vi "SingleLayerReport.vi"(0 "IP address":string="192.168.1.214", 5 "LayerID under test":u32 format="%x", 7 "All ID list":u32[](array[numeric]) format="%x", 9 "Report folder path":path, 11 "process":string) -> (4 "Layer Report file path":path, 8 "Test OK?":bool, 10 "Report out":string, 15 "error out":errorcluster)   [LabVIEW 2015, in "VIPM2.lvlib"]
uses:
  VIPM2.lvlib
panel:
  in  "TDCValues":i32=5
  out "STATUS MONITOR":string="CLOSING TCP/IP CONNECTION"
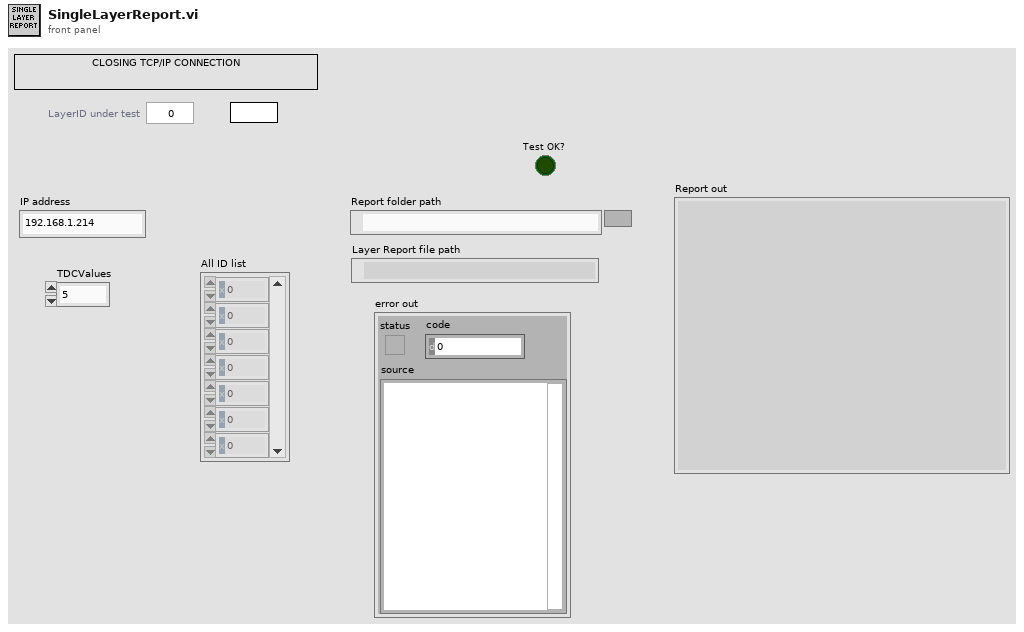
[diagram p1: front panel]
types:
  T1 = enum16{"open", "replace", "create", "open or create", "replace or create", "replace or create with confirmation"}
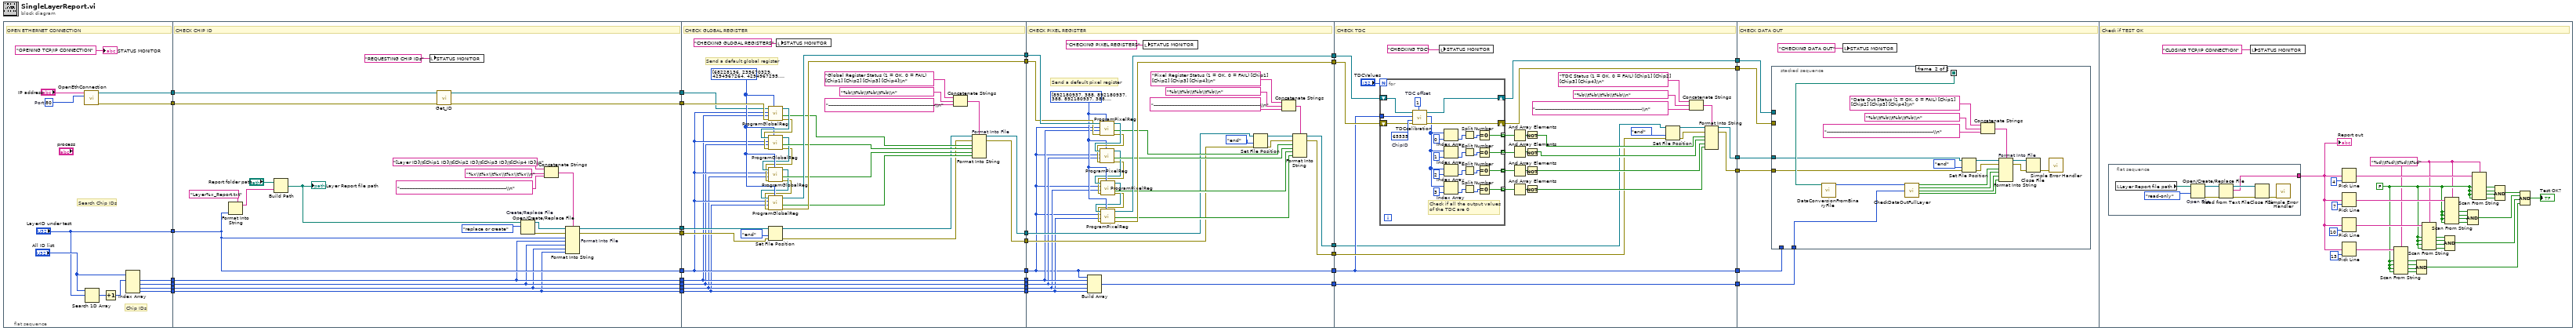
[diagram p0: block diagram]
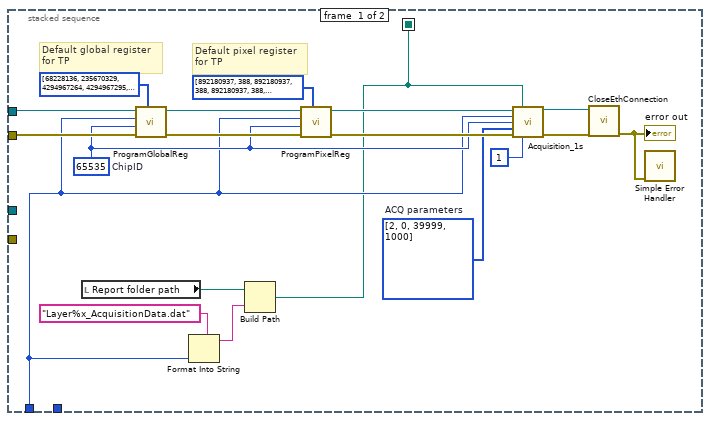
[diagram p2: hidden frame]
diagram:
  n1 = flat-sequence {
    tunnel: [w47] -> w7
    tunnel: [w46] -> w6
    tunnel: ["LayerID under test"] -> w5
    tunnel: [w41] -> w4
    tunnel: [w40] -> w3
    tunnel: [w39] -> w2
    tunnel: [w38] -> w1
    tunnel: w7 -> [w54]
    tunnel: [w52] -> w37
    tunnel: w6 -> [w53]
    tunnel: [w51] -> w36
    tunnel: [w59] -> w29
    tunnel: [w58] -> w28
    tunnel: [w57] -> w27
    tunnel: [w56] -> w26
    tunnel: [w55] -> w25
    tunnel: [w61] -> w24
    tunnel: [w60] -> w23
    tunnel: w5 -> [w59]
    tunnel: w4 -> [w58]
    tunnel: w3 -> [w57]
    tunnel: w2 -> [w56]
    tunnel: w1 -> [w55]
    tunnel: w37 -> [w85]
    tunnel: [w105] -> w35
    tunnel: w36 -> [w104]
    tunnel: [w103] -> w34
    tunnel: w29 -> [w80]
    tunnel: w28 -> [w79]
    tunnel: w27 -> [w78]
    tunnel: w26 -> [w77]
    tunnel: w25 -> [w76]
    tunnel: w24 -> [w84]
    tunnel: w23 -> [w83]
    tunnel: [w80] -> w22
    tunnel: [w79] -> w21
    tunnel: [w78] -> w20
    tunnel: [w77] -> w19
    tunnel: [w76] -> w18
    tunnel: [w75] -> w17
    tunnel: [w74] -> w16
    tunnel: w35 -> [w138]
    tunnel: [w137] -> w33
    tunnel: w34 -> [w134]
    tunnel: [w136] -> w32
    tunnel: w22 -> [w106]
    tunnel: w21 -> [w111]
    tunnel: w20 -> [w110]
    tunnel: w19 -> [w109]
    tunnel: w18 -> [w108]
    tunnel: w17 -> [w115]
    tunnel: w16 -> [w114]
    tunnel: [w106] -> w15
    tunnel: [w113] -> w14
    tunnel: [w112] -> w13
    tunnel: [w107] -> w9
    tunnel: w33 -> [w169]
    tunnel: [w168] -> w31
    tunnel: w32 -> [w167]
    tunnel: [w166] -> w30
    tunnel: w15 -> [w143]
    tunnel: w14 -> [w142]
    tunnel: w13 -> [w144]
    tunnel: [w143] -> w12
    tunnel: [w141] -> w11
    tunnel: [w140] -> w10
    tunnel: w9 -> [w139]
    tunnel: [w139] -> w8
    tunnel: w31 -> [w197]
    tunnel: w30 -> [w199]
    tunnel: w12 -> [w198]
    tunnel: w11 -> [w196]
    tunnel: w10 -> [w195]
    tunnel: w8 -> [w194]
    frame #0 {
      w49 = u16 80  # Port
      # "Chip IDs"
      # "Search Chip IDs"
      # "OPEN ETHERNET CONNECTION"
      n2 = call "OpenEthConnection.vi"("Port"=w49, "IP address"="IP address") -> ("error out"=w46:errorcluster, "connection ID out"=w47:refnum<k5>)  [unwired: 7 in, 1 out]
      n3 = Search 1D Array(1D array="All ID list", element="LayerID under test") -> (index of element=w44:i32)  [unwired: 1 in]
      n4 = Increment(x=w44) -> (x+1=w45:i32)
      n5 = Index Array "Index Array"(array="All ID list", index #1=w45) -> (element #1=w41:u32, element #2=w40:u32, element #3=w39:u32, element #4=w38:u32)  [unwired: 3 in]
      "STATUS MONITOR" <- "OPENING TCP/IP CONNECTION" ("STATUS MONITOR")
    }
    frame #1 {
      # "CHECK CHIP ID"
      n6 = Format Into String(format string="Layer%x_Report.txt", w59) -> (resulting string=w63:string)  [unwired: 2 in, 1 out]
      n7 = Build Path(base path="Report folder path", name or relative path=w63) -> (appended path=w72:path)
      "Layer Report file path" <- w72
      n8 = local write "STATUS MONITOR"("REQUESTING CHIP IDs" ("STATUS MONITOR")) -> ()
      n9 = call "Get_ID.vi"("error in (no error)"=w53, "connection ID"=w54) -> ("error out"=w51:errorcluster, "connection ID out"=w52:refnum<k5>)  [unwired: 6 in, 2 out]
      n10 = Open/Create/Replace File "Create/Replace File"(file path (use dialog)=w72, operation (0:open)=T1."replace or create") -> (refnum out=w70:refnum<file>, error out=w65:errorcluster)  [unwired: 4 in, 1 out]
      n11 = Concatenate Strings "Concatenate Strings"("[Layer ID]\\t[Chip1 ID]\\t[Chip2 ID]\\t[Chip3 ID]\\t[Chip4 ID]\\n" ("format string"), "%x\\t%x\\t%x\\t%x\\t%x\\n" ("format string"), "--------------------------------------------------------------------\\n" ("format string")) -> (w66:string)
      n12 = Format Into String "Format Into File"(format string=w66, initial string=w70, error in=w65, w59, w58, w57, w56, w55) -> (resulting string=w61:refnum<file>, error out=w60:errorcluster)
    }
    frame #2 {
      w90 = u32[] [68228136, 235670329, 4294967264, 4294967295, 4294967295, 511] ("DefaultGlobal Reg_TP")
      # "Send a default global register"
      # "CHECK GLOBAL REGISTER"
      n13 = call "ProgramGlobalReg.vi"("Global Reg"=w90, "error in (no error)"=w104, "ChipID"=w79, "LayerID"=w80, "connection ID"=w85) -> ("error out"=w93:errorcluster, "OK?"=w91:bool, "connection ID out"=w101:refnum<k5>)  [unwired: 2 in, 2 out]
      n14 = call "ProgramGlobalReg.vi"("Global Reg"=w90, "error in (no error)"=w93, "ChipID"=w78, "LayerID"=w80, "connection ID"=w101) -> ("error out"=w87:errorcluster, "OK?"=w96:bool, "connection ID out"=w89:refnum<k5>)  [unwired: 2 in, 2 out]
      n15 = Set File Position(refnum=w84, from (0:start)=enum16{"start", "end", "current"}."end", error in=w83) -> (refnum out=w82:refnum<file>, error out=w81:errorcluster)  [unwired: 1 in]
      n16 = call "ProgramGlobalReg.vi"("Global Reg"=w90, "error in (no error)"=w87, "ChipID"=w77, "LayerID"=w80, "connection ID"=w89) -> ("error out"=w86:errorcluster, "OK?"=w95:bool, "connection ID out"=w88:refnum<k5>)  [unwired: 2 in, 2 out]
      n17 = call "ProgramGlobalReg.vi"("Global Reg"=w90, "error in (no error)"=w86, "ChipID"=w76, "LayerID"=w80, "connection ID"=w88) -> ("error out"=w103:errorcluster, "OK?"=w94:bool, "connection ID out"=w105:refnum<k5>)  [unwired: 2 in, 2 out]
      n18 = local write "STATUS MONITOR"("CHECKING GLOGAL REGISTERS" ("STATUS MONITOR")) -> ()
      n19 = Concatenate Strings "Concatenate Strings"("Global Register Status (1 = OK, 0 = FAIL) [Chip1] [Chip2] [Chip3] [Chip4]\\n" ("format string"), "%b\\t%b\\t%b\\t%b\\n" ("format string"), "--------------------------------------------------------------------\\n" ("format string")) -> (w99:string)
      n20 = Format Into String "Format Into File"(format string=w99, initial string=w82, error in=w81, w91, w96, w95, w94) -> (resulting string=w75:refnum<file>, error out=w74:errorcluster)
    }
    frame #3 {
      w121 = u32[] [892180937, 388, 892180937, 388, 892180937, 388, 892180937, 388, 892180937, 388, 892180937, 388, 892180937, 388, 892180937, 388, 892180937, 388, 892180937, 388, 892180937, 388, 892180937, 388, 892180937, 388, 892180937, 388, 892180937, 388, 892180937, 388, 892180937, 388, 892180937, 388, 892180937, 388, 892180937, 388, 892180937, 388, 892180937, 388, 892180937, 388, 892180937, 388, 892180937, 388, 892180937, 388, 892180937, 388, 892180937, 388, 892180937, 388, 892180937, 388, 892180937, 388, 892180937, 388, 892180937, 388, 1092475113, 180, 892180937, 388, 892180937, 388, 892180937, 388, 892180937, 388, 892180937, 388, 892180937, 388, 892180937, 388, 892180937, 388, 892180937, 388, 892180937, 388, 892180937, 388, 892180937, 388, 892180937, 388, 892180937, 388, 892180937, 388, 892180937, 388, 892180937, 388, 892180937, 388, 892180937, 388, 892180937, 388, 892180937, 388, 892180937, 388, 892180937, 388, 892180937, 388, 892180937, 388, 892180937, 388, 892180937, 388, 892180937, 388, 892180937, 388, 892180937, 388, 892180937, 388, 892180937, 388, 892180937, 388, 892180937, 388, 892180937, 388, 892180937, 388, 892180937, 388, 892180937, 388, 892180937, 388, 892180937, 388, 892180937, 388, 892180937, 388, 892180937, 388, 892180937, 388, 892180937, 388, 892180937, 388, 892180937, 388, 892180937, 388, 892180937, 388, 892180937, 388, 892180937, 388, 892180937, 388, 892180937, 388, 892180937, 388, 892180937, 388, 892180937, 388, 892180937, 388, 892180937, 388, 892180937, 388, 892180937, 388, 892180937, 388, 892180937, 388, 892180937, 388, 892180937, 388, 892180937, 388, 892180937, 388] ("DefaultPixel Register Array_TP")
      # "Send a default pixel register"
      # "CHECK PIXEL REGISTER"
      n21 = Build Array "Build Array"(w106, w111, w110, w109, w108) -> (w107:u32[])
      n22 = call "ProgramPixelReg.vi"("Pixel Register"=w121, "error in (no error)"=w134, "ChipID"=w111, "LayerID"=w106, "connection ID"=w138) -> ("error out"=w126:errorcluster, "OK?"=w122:bool, "connection ID out"=w133:refnum<k5>)  [unwired: 2 in, 2 out]
      n23 = call "ProgramPixelReg.vi"("Pixel Register"=w121, "error in (no error)"=w126, "ChipID"=w110, "LayerID"=w106, "connection ID"=w133) -> ("error out"=w118:errorcluster, "OK?"=w129:bool, "connection ID out"=w120:refnum<k5>)  [unwired: 2 in, 2 out]
      n24 = call "ProgramPixelReg.vi"("Pixel Register"=w121, "error in (no error)"=w118, "ChipID"=w109, "LayerID"=w106, "connection ID"=w120) -> ("error out"=w117:errorcluster, "OK?"=w128:bool, "connection ID out"=w119:refnum<k5>)  [unwired: 2 in, 2 out]
      n25 = call "ProgramPixelReg.vi"("Pixel Register"=w121, "error in (no error)"=w117, "ChipID"=w108, "LayerID"=w106, "connection ID"=w119) -> ("error out"=w136:errorcluster, "OK?"=w127:bool, "connection ID out"=w137:refnum<k5>)  [unwired: 2 in, 2 out]
      n26 = local write "STATUS MONITOR"("CHECKING PIXEL REGISTERS" ("STATUS MONITOR")) -> ()
      n27 = Set File Position(refnum=w115, from (0:start)=enum16{"start", "end", "current"}."end", error in=w114) -> (refnum out=w124:refnum<file>, error out=w116:errorcluster)  [unwired: 1 in]
      n28 = Concatenate Strings("Pixel Register Status (1 = OK, 0 = FAIL) [Chip1] [Chip2] [Chip3] [Chip4]\\n" ("format string"), "%b\\t%b\\t%b\\t%b\\n" ("format string"), "--------------------------------------------------------------------\\n" ("format string")) -> (w123:string)
      n29 = Format Into String(format string=w123, initial string=w124, error in=w116, w122, w129, w128, w127) -> (resulting string=w113:refnum<file>, error out=w112:errorcluster)
    }
    frame #4 {
      # "CHECK TDC"
      n30 = for {
        N: "TDCValues" -> [_]
        tunnel: w143 -> [w192]
        shift-right: [w189] -> w166
        shift-left: w167 -> [w190]
        shift-right: [w170] -> w168
        shift-left: w169 -> [w171]
        tunnel: [w175] -> w163 mode=indexing
        tunnel: [w174] -> w162 mode=indexing
        tunnel: [w173] -> w161 mode=indexing
        tunnel: [w172] -> w160 mode=indexing
        w191 = u32 65535  # ChipID
        w193 = u32 1  # TDC offset
        # "Check if all the output values\nof the TDC are 0"
        n31 = call "TDCcalibration.vi"("TDC offset"=w193, "error in (no error)"=w190, "ChipID"=w191, "LayerID"=w192, "connection ID"=w171) -> ("error out"=w189:errorcluster, "TDC calibration data"=w188:u32[], "connection ID out"=w170:refnum<k5>)  [unwired: 3 in, 1 out]
        n32 = Index Array(array=w188, index=0) -> (element=w183:u32)
        n33 = Index Array(array=w188, index=1) -> (element=w178:u32)
        n34 = Index Array(array=w188, index=2) -> (element=w177:u32)
        n35 = Index Array(array=w188, index=3) -> (element=w176:u32)
        n36 = Split Number(x=w183) -> (lo(x)=w182:u16)  [unwired: 1 out]
        n37 = Split Number(x=w178) -> (lo(x)=w181:u16)  [unwired: 1 out]
        n38 = Split Number(x=w177) -> (lo(x)=w180:u16)  [unwired: 1 out]
        n39 = Split Number(x=w176) -> (lo(x)=w179:u16)  [unwired: 1 out]
        n40 = Equal To 0?(x=w182) -> (x = 0?=w175:bool)
        n41 = Equal To 0?(x=w181) -> (x = 0?=w174:bool)
        n42 = Equal To 0?(x=w180) -> (x = 0?=w173:bool)
        n43 = Equal To 0?(x=w179) -> (x = 0?=w172:bool)
      }
      n44 = local write "STATUS MONITOR"("CHECKING TDC" ("STATUS MONITOR")) -> ()
      n45 = And Array Elements(Boolean array=w163) -> (logical AND=w154:bool)
      n46 = And Array Elements(Boolean array=w162) -> (logical AND=w153:bool)
      n47 = And Array Elements(Boolean array=w161) -> (logical AND=w152:bool)
      n48 = And Array Elements(Boolean array=w160) -> (logical AND=w151:bool)
      n49 = Not(x=w154) -> (.not. x?=w150:bool)
      n50 = Not(x=w153) -> (.not. x?=w149:bool)
      n51 = Not(x=w152) -> (.not. x?=w148:bool)
      n52 = Not(x=w151) -> (.not. x?=w147:bool)
      n53 = Set File Position(refnum=w142, from (0:start)=enum16{"start", "end", "current"}."end", error in=w144) -> (refnum out=w156:refnum<file>, error out=w146:errorcluster)  [unwired: 1 in]
      n54 = Concatenate Strings("TDC Status (1 = OK, 0 = FAIL) [Chip1] [Chip2] [Chip3] [Chip4]\\n" ("format string"), "%b\\t%b\\t%b\\t%b\\n" ("format string"), "--------------------------------------------------------------------\\n" ("format string")) -> (w155:string)
      n55 = Format Into String(format string=w155, initial string=w156, error in=w146, w150, w149, w148, w147) -> (resulting string=w141:refnum<file>, error out=w140:errorcluster)
    }
    frame #5 {
      # "CHECK DATA OUT"
      n56 = stacked-sequence {
        seq-local: [w204 _] -> [_ w223]
        tunnel: w199 -> [w219 _]
        tunnel: w198 -> [w205 _]
        tunnel: w197 -> [w209 _]
        tunnel: w195 -> [_ w222]
        tunnel: w196 -> [_ w221]
        tunnel: w194 -> [_ w220]
        frame #0 {
          w211 = u32[] [2, 0, 39999, 1000]  # ACQ parameters
          w212 = u32 65535  # ChipID
          # "Default pixel register \nfor TP"
          # "Default global register \nfor TP"
          n57 = local read "Report folder path"() -> (w207:path)
          n58 = call "ProgramGlobalReg.vi"("Global Reg"=u32[] [68228136, 235670329, 4294967264, 4294967295, 4294967295, 511] ("DefaultGlobal Reg_TP"), "error in (no error)"=w219, "ChipID"=w212, "LayerID"=w205, "connection ID"=w209) -> ("error out"=w216:errorcluster, "connection ID out"=w217:refnum<k5>)  [unwired: 2 in, 3 out]
          n59 = Format Into String(format string="Layer%x_AcquisitionData.dat", w205) -> (resulting string=w206:string)  [unwired: 2 in, 1 out]
          n60 = Build Path(base path=w207, name or relative path=w206) -> (appended path=w204:path)
          n61 = call "ProgramPixelReg.vi"("Pixel Register"=u32[] [892180937, 388, 892180937, 388, 892180937, 388, 892180937, 388, 892180937, 388, 892180937, 388, 892180937, 388, 892180937, 388, 892180937, 388, 892180937, 388, 892180937, 388, 892180937, 388, 892180937, 388, 892180937, 388, 892180937, 388, 892180937, 388, 892180937, 388, 892180937, 388, 892180937, 388, 892180937, 388, 892180937, 388, 892180937, 388, 892180937, 388, 892180937, 388, 892180937, 388, 892180937, 388, 892180937, 388, 892180937, 388, 892180937, 388, 892180937, 388, 892180937, 388, 892180937, 388, 892180937, 388, 1092475113, 180, 892180937, 388, 892180937, 388, 892180937, 388, 892180937, 388, 892180937, 388, 892180937, 388, 892180937, 388, 892180937, 388, 892180937, 388, 892180937, 388, 892180937, 388, 892180937, 388, 892180937, 388, 892180937, 388, 892180937, 388, 892180937, 388, 892180937, 388, 892180937, 388, 892180937, 388, 892180937, 388, 892180937, 388, 892180937, 388, 892180937, 388, 892180937, 388, 892180937, 388, 892180937, 388, 892180937, 388, 892180937, 388, 892180937, 388, 892180937, 388, 892180937, 388, 892180937, 388, 892180937, 388, 892180937, 388, 892180937, 388, 892180937, 388, 892180937, 388, 892180937, 388, 892180937, 388, 892180937, 388, 892180937, 388, 892180937, 388, 892180937, 388, 892180937, 388, 892180937, 388, 892180937, 388, 892180937, 388, 892180937, 388, 892180937, 388, 892180937, 388, 892180937, 388, 892180937, 388, 892180937, 388, 892180937, 388, 892180937, 388, 892180937, 388, 892180937, 388, 892180937, 388, 892180937, 388, 892180937, 388, 892180937, 388, 892180937, 388, 892180937, 388, 892180937, 388, 892180937, 388, 892180937, 388] ("DefaultPixel Register Array_TP"), "error in (no error)"=w216, "ChipID"=w212, "LayerID"=w205, "connection ID"=w217) -> ("error out"=w214:errorcluster, "connection ID out"=w213:refnum<k5>)  [unwired: 2 in, 3 out]
          n62 = call "Acquisition_1s.vi"("connection ID"=w213, "File ACQ data"=w204, "LayerID"=w205, "ChipID"=w212, "ACQ parameters"=w211, "error in (no error)"=w214, "Acquisition time (s)"=u32 1) -> ("connection ID out"=w203:refnum<k5>, "error out"=w202:errorcluster)  [unwired: 4 in, 3 out]
          n63 = call "CloseEthConnection.vi"("error in (no error)"=w202, "connection ID"=w203) -> ("error out"=w201:errorcluster)  [unwired: 9 in]
          "error out" <- w201
          n64 = call <vilib>:"Simple Error Handler.vi"("error in (no error)"=w201) -> ()  [unwired: 4 in, 5 out]
        }
        frame #1 {
          n65 = call "DataConversionFromBinaryFile.vi"("file (use dialog)"=w223) -> ("Output Array"=w238:u32[])  [unwired: 8 in]
          n66 = call "CheckDataOutFullLayer.vi"("InputEventWord"=w238, "ID list"=w220) -> ("DataChip1 OK?"=w230:bool, "DataChip2 OK?"=w229:bool, "DataChip3 OK?"=w228:bool, "DataChip4 OK?"=w227:bool)  [unwired: 10 in]
          n67 = Set File Position(refnum=w221, from (0:start)=enum16{"start", "end", "current"}."end", error in=w222) -> (refnum out=w232:refnum<file>, error out=w226:errorcluster)  [unwired: 1 in]
          n68 = Concatenate Strings "Concatenate Strings"("Data Out Status (1 = OK, 0 = FAIL) [Chip1] [Chip2] [Chip3] [Chip4]\\n" ("format string"), "%b\\t%b\\t%b\\t%b\\n" ("format string"), "--------------------------------------------------------------------\\n" ("format string")) -> (w231:string)
          n69 = Format Into String "Format Into File"(format string=w231, initial string=w232, error in=w226, w230, w229, w228, w227) -> (resulting string=w234:refnum<file>, error out=w225:errorcluster)
          n70 = Close File(refnum=w234, error in=w225) -> (error out=w224:errorcluster)  [unwired: 1 out]
          n71 = call <vilib>:"Simple Error Handler.vi"("error in (no error)"=w224) -> ()  [unwired: 4 in, 5 out]
        }
      }
      n72 = local write "STATUS MONITOR"("CHECKING DATA OUT" ("STATUS MONITOR")) -> ()
    }
    frame #6 {
      w245 = FALSE
      w239 = "%d\\t%d\\t%d\\t%d" ("format string")
      # "Check if TEST OK"
      n73 = flat-sequence {
        tunnel: [w272] -> w266
        frame #0 {
          n74 = local read "Layer Report file path"() -> (w279:path)
          n75 = Open/Create/Replace File "Open File"(file path (use dialog)=w279, access (0:read/write)=enum16{"read/write", "read-only", "write-only"}."read-only") -> (refnum out=w277:refnum<file>, error out=w276:errorcluster)  [unwired: 4 in, 1 out]
          n76 = Read from Text File(file (use dialog)=w277, error in=w276) -> (refnum out=w275:refnum<file>, text=w272:string, error out=w274:errorcluster)  [unwired: 2 in, 1 out]
          n77 = Close File(refnum=w275, error in=w274) -> (error out=w273:errorcluster)  [unwired: 1 out]
          n78 = call <vilib>:"Simple Error Handler.vi"("error in (no error)"=w273) -> ()  [unwired: 4 in, 5 out]
        }
      }
      n79 = local write "STATUS MONITOR"("CLOSING TCP/IP CONNECTION" ("STATUS MONITOR")) -> ()
      n80 = Pick Line(multi-line string=w266, line index=4) -> (output string=w246:string)  [unwired: 1 in]
      n81 = Pick Line(multi-line string=w266, line index=7) -> (output string=w257:string)  [unwired: 1 in]
      n82 = Pick Line(multi-line string=w266, line index=10) -> (output string=w252:string)  [unwired: 1 in]
      n83 = Pick Line(multi-line string=w266, line index=13) -> (output string=w247:string)  [unwired: 1 in]
      n84 = Scan From String(format string=w239, input string=w247, default 1=w245, default 2=w245, default 3=w245, default 4=w245) -> (output 1=w248:bool, output 2=w249:bool, output 3=w250:bool, output 4=w251:bool)  [unwired: 2 in, 3 out]
      n85 = Compound Arithmetic op=AND(w248, w249, w250, w251) -> (w240:bool)
      n86 = Scan From String(format string=w239, input string=w252, default 1=w245, default 2=w245, default 3=w245, default 4=w245) -> (output 1=w256:bool, output 2=w255:bool, output 3=w254:bool, output 4=w253:bool)  [unwired: 2 in, 3 out]
      n87 = Compound Arithmetic op=AND(w256, w255, w254, w253) -> (w241:bool)
      n88 = Scan From String(format string=w239, input string=w257, default 1=w245, default 2=w245, default 3=w245, default 4=w245) -> (output 1=w258:bool, output 2=w259:bool, output 3=w260:bool, output 4=w261:bool)  [unwired: 2 in, 3 out]
      n89 = Compound Arithmetic op=AND(w258, w259, w260, w261) -> (w242:bool)
      n90 = Scan From String(format string=w239, input string=w246, default 1=w245, default 2=w245, default 3=w245, default 4=w245) -> (output 1=w265:bool, output 2=w264:bool, output 3=w263:bool, output 4=w262:bool)  [unwired: 2 in, 3 out]
      n91 = Compound Arithmetic op=AND(w265, w264, w263, w262) -> (w243:bool)
      n92 = Compound Arithmetic op=AND(w243, w242, w241, w240) -> (→"Test OK?":bool)
      "Report out" <- w266
    }
  }
